vi "BuildHMatrix.vi"(8 "error in (no error)":errorcluster, 9 "Z":dbl[](array[numeric]), 10 "Y":dbl[](array[numeric]), 11 "X":dbl[](array[numeric])) -> (0 "error out":errorcluster, 1 "terms":string[](array[string]), 2 "H":dbl[][](array[numeric]))   [LabVIEW 2023, in "Utilities.lvclass"]
uses:
  Utilities.lvclass
panel:
  in  "Highest order":i32=3
  out "Utilities out":refnum<class "Utilities.lvclass">
  in  "Utilities in":refnum<class "Utilities.lvclass">
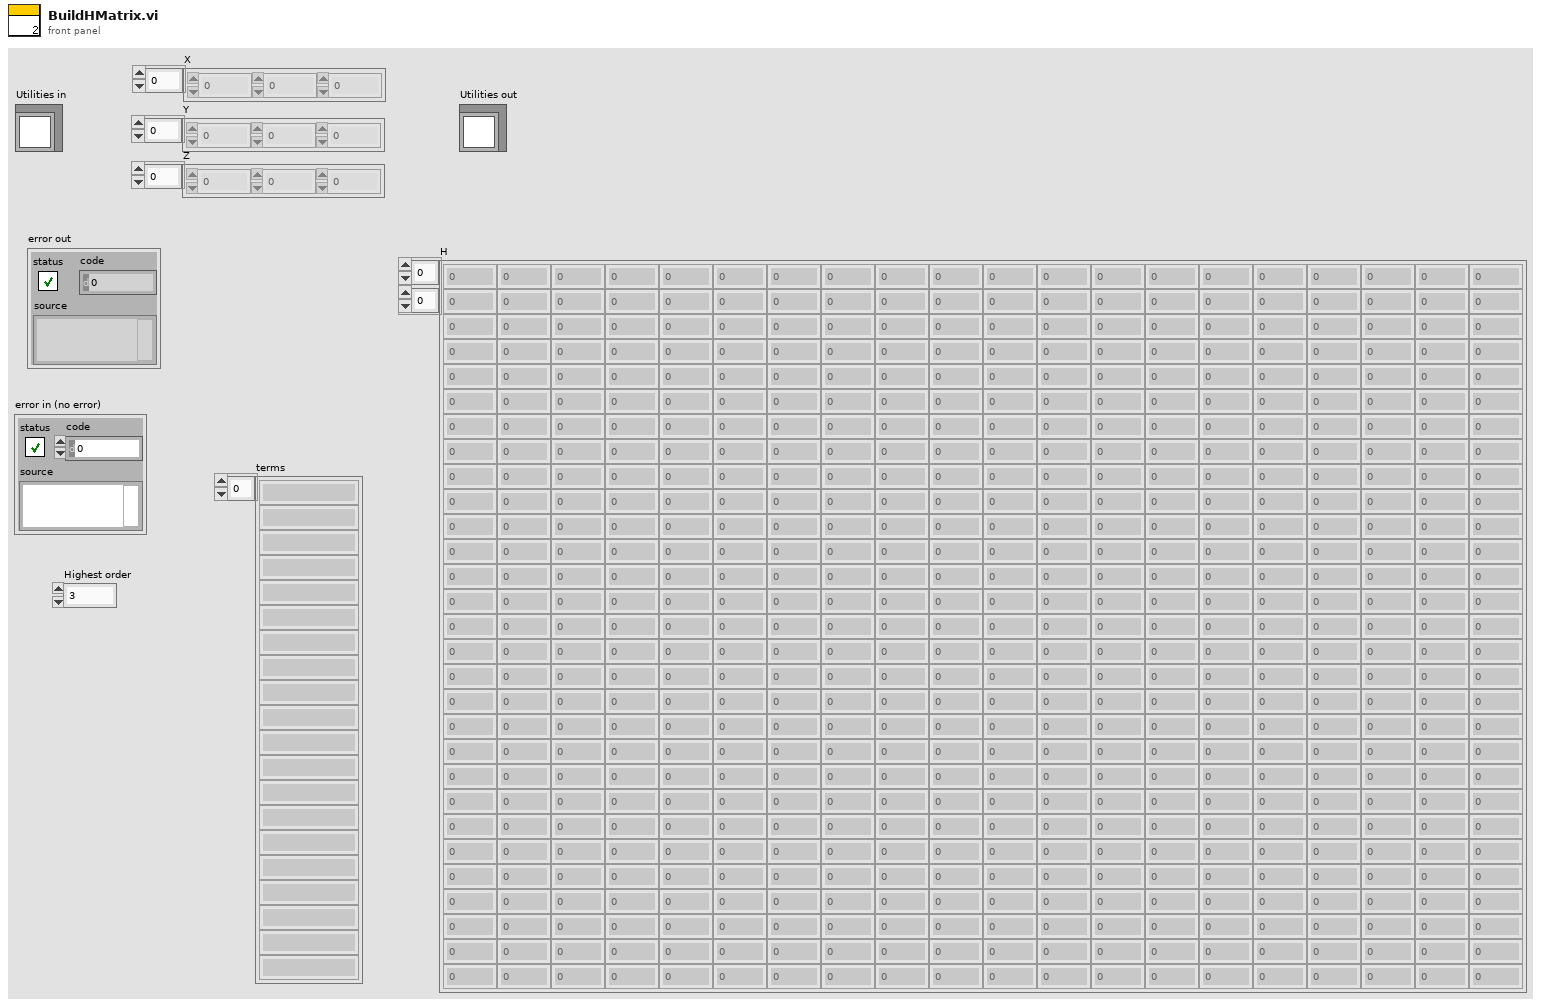
[diagram p1: front panel]
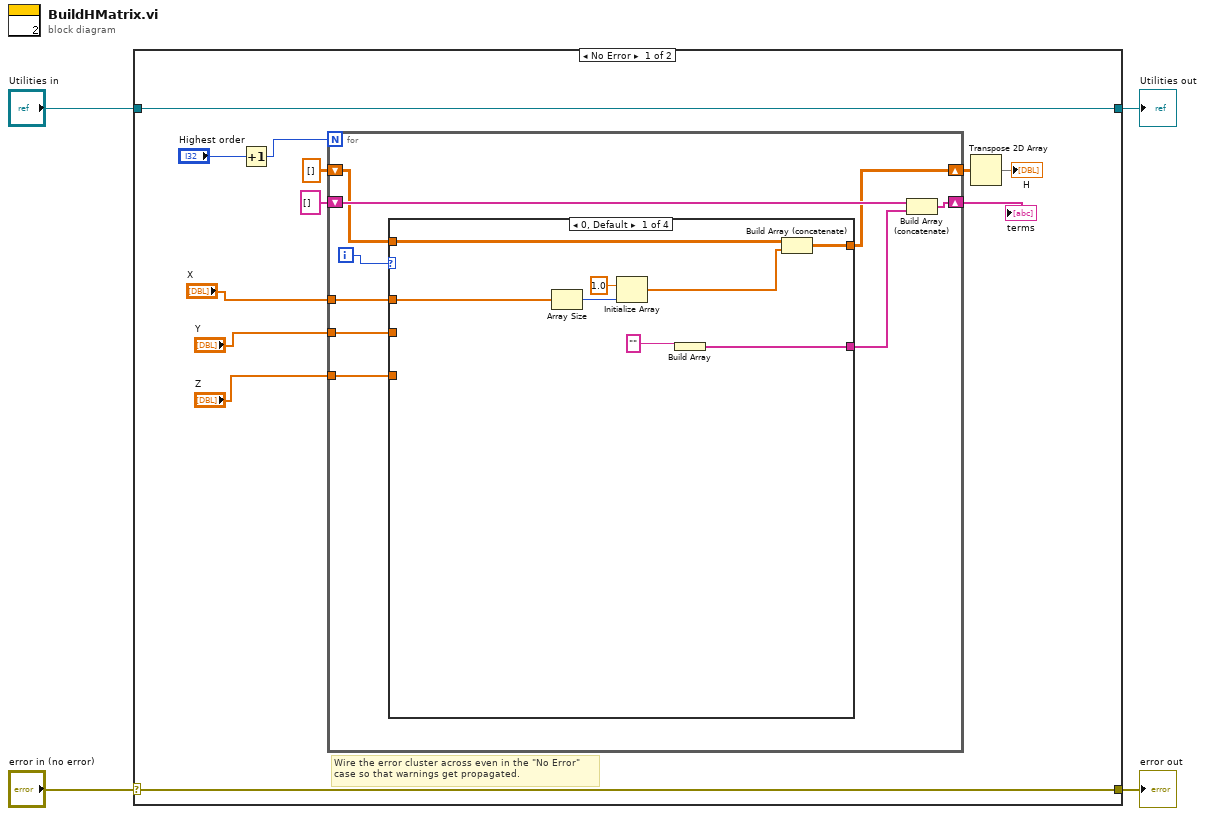
[diagram p0: block diagram]
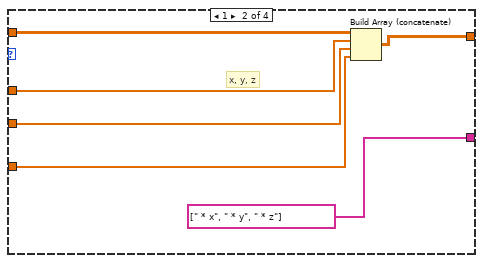
[diagram p2: hidden frame]
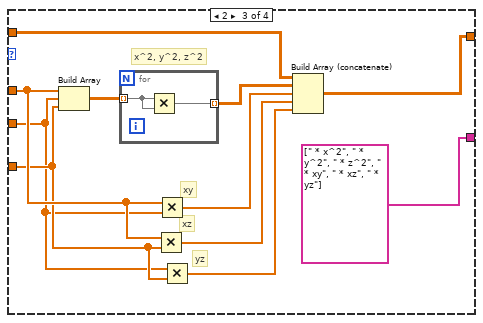
[diagram p3: hidden frame]
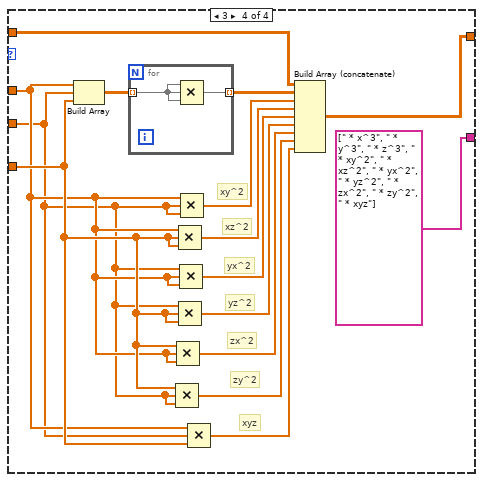
[diagram p4: hidden frame]
diagram:
  n1 = case shown="No Error" "error in (no error)" {
    selector: "error in (no error)" -> [w15 w71]
    tunnel: [w15 w71] -> w3
    tunnel: [w16 w70] -> w1
    tunnel: "Utilities in" -> [w16 w70]
    frame No Error {
      # "Wire the error cluster across even in the \"No Error\"\ncase so that warnings get propagated."
      n2 = Increment(x="Highest order") -> (x+1=w8:i32)
      n3 = for {
        N: w8 -> [_]
        tunnel: "X" -> [w21]
        tunnel: "Y" -> [w20]
        shift-right: [w17] -> w14
        shift-left: dbl[][] [] ("transposed array") -> [w18]
        shift-right: [w24] -> w10
        shift-left: string[] [] -> [w25]
        tunnel: "Z" -> [w19]
        i -> [w23]
        n4 = case shown="0, Default" w23 {
          tunnel: [w32 string[] [" * x", " * y", " * z"] string[] [" * x^2", " * y^2", " * z^2", " * xy", " * xz", " * yz"] ("Array 2") string[] [" * x^3", " * y^3", " * z^3", " * xy^2", " * xz^2", " * yx^2", " * yz^2", " * zx^2", " * zy^2", " * xyz"] ("Array 2")] -> w22
          tunnel: w21 -> [w31 w38 w47 w55]
          tunnel: w20 -> [_ w37 w45 w54]
          tunnel: w19 -> [_ w36 w46 w56]
          tunnel: w18 -> [w28 w39 w49 w53]
          tunnel: [w26 w35 w41 w67] -> w17
          frame 0, Default {
            n5 = Array Size(array=w31) -> (size(s)=w30:i32)
            n6 = Initialize Array(1.0 ("element"), w30) -> (w27:dbl[])
            n7 = Build Array("" ("format string")) -> (w32:string[])
            n8 = Build Array (concatenate)(w28, w27) -> (w26:dbl[][])
          }
          frame 1 {
            # "x, y, z"
            n9 = Build Array (concatenate)(w39, w38, w37, w36) -> (w35:dbl[][])
          }
          frame 2 {
            # "yz"
            # "xz"
            # "xy"
            # "x^2, y^2, z^2"
            n10 = Build Array(w47, w45, w46) -> (w50:dbl[][])
            n11 = for {
              tunnel: w50 -> [w52] mode=indexing
              tunnel: [w51] -> w48 mode=indexing
              n12 = Multiply(x=w52, y=w52) -> (x*y=w51:dbl[])
            }
            n13 = Multiply(x=w47, y=w46) -> (x*y=w43:dbl[])
            n14 = Multiply(x=w47, y=w45) -> (x*y=w44:dbl[])
            n15 = Multiply(x=w45, y=w46) -> (x*y=w42:dbl[])
            n16 = Build Array (concatenate)(w49, w48, w44, w43, w42) -> (w41:dbl[][])
          }
          frame 3 {
            # "xyz"
            # "zy^2"
            # "zx^2"
            # "yz^2"
            # "yx^2"
            # "xz^2"
            # "xy^2"
            n17 = Build Array(w55, w54, w56) -> (w66:dbl[][])
            n18 = for {
              tunnel: w66 -> [w69] mode=indexing
              tunnel: [w68] -> w59 mode=indexing
              n19 = Compound Arithmetic op=MULTIPLY(w69, w69, w69) -> (w68:dbl[])
            }
            n20 = Compound Arithmetic op=MULTIPLY(w56, w54, w54) -> (w63:dbl[])
            n21 = Compound Arithmetic op=MULTIPLY(w56, w55, w55) -> (w62:dbl[])
            n22 = Compound Arithmetic op=MULTIPLY(w55, w56, w56) -> (w58:dbl[])
            n23 = Compound Arithmetic op=MULTIPLY(w54, w56, w56) -> (w61:dbl[])
            n24 = Compound Arithmetic op=MULTIPLY(w54, w55, w55) -> (w60:dbl[])
            n25 = Compound Arithmetic op=MULTIPLY(w55, w54, w54) -> (w57:dbl[])
            n26 = Compound Arithmetic op=MULTIPLY(w55, w54, w56) -> (w64:dbl[])
            n27 = Build Array (concatenate)(w53, w59, w57, w58, w60, w61, w62, w63, w64) -> (w67:dbl[][])
          }
        }
        n28 = Build Array (concatenate)(w25, w22) -> (w24:string[])
      }
      "terms" <- w10
      n29 = Transpose 2D Array(2D array=w14) -> (transposed array=→"H":dbl[][])
    }
    frame Error {
    }
  }
  "error out" <- w3
  "Utilities out" <- w1
